vi "mWADC_FreqToRev.vi"(9 "Intercept":dbl, 10 "Slope":dbl, 11 "Frequecy":dbl) -> (3 "Revolutions":dbl)   [LabVIEW 2019]
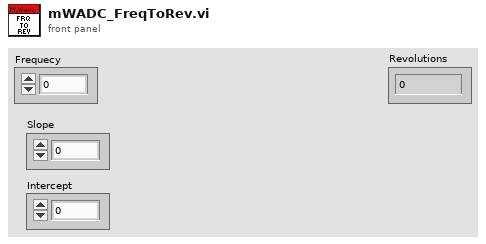
[diagram p1: front panel]
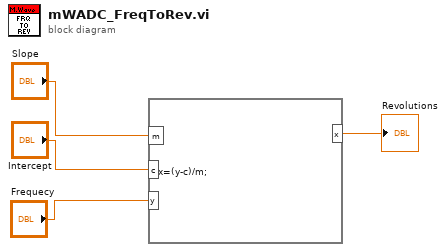
[diagram p0: block diagram]
diagram:
  n1 = formula code="x=(y-c)/m;"("m"="Slope", "c"="Intercept", "y"="Frequecy") -> ("x"=→"Revolutions":dbl)
